vi "data logging.vi"   [LabVIEW 2017]
uses:
  Robot Global Data.vi
  <vilib>/Utility/file.llb/Write Delimited Spreadsheet (string).vi
types:
  T1 = typedef "WPI_EncoderDevRef.ctl" = cluster{"DevStatus":errorcluster, "EncoderIndex":T2, "CounterIndex":T3, "DistancePerCount":dbl, "Decoding Type":T4}
  T2 = typedef "FPGA_EncoderIdx.ctl" = enum8{"Enc 0", "Enc 1", "Enc 2", "Enc 3", "Enc 4", "Enc 5", "Enc 6", "Enc 7", "Invalid"}
  T3 = typedef "FPGA_CounterCtrSystemIndex.ctl" = enum8{"Ctr 0", "Ctr 1", "Ctr 2", "Ctr 3", "Ctr 4", "Ctr 5", "Ctr 6", "Ctr 7", "Invalid"}
  T4 = typedef "WPI_EncoderType.ctl" = enum16{"1x", "2x", "4x"}
  T5 = cluster{"Yaw":dbl, "Roll":dbl, "Pitch":dbl, "Heading":dbl, "Fused Heading":dbl}
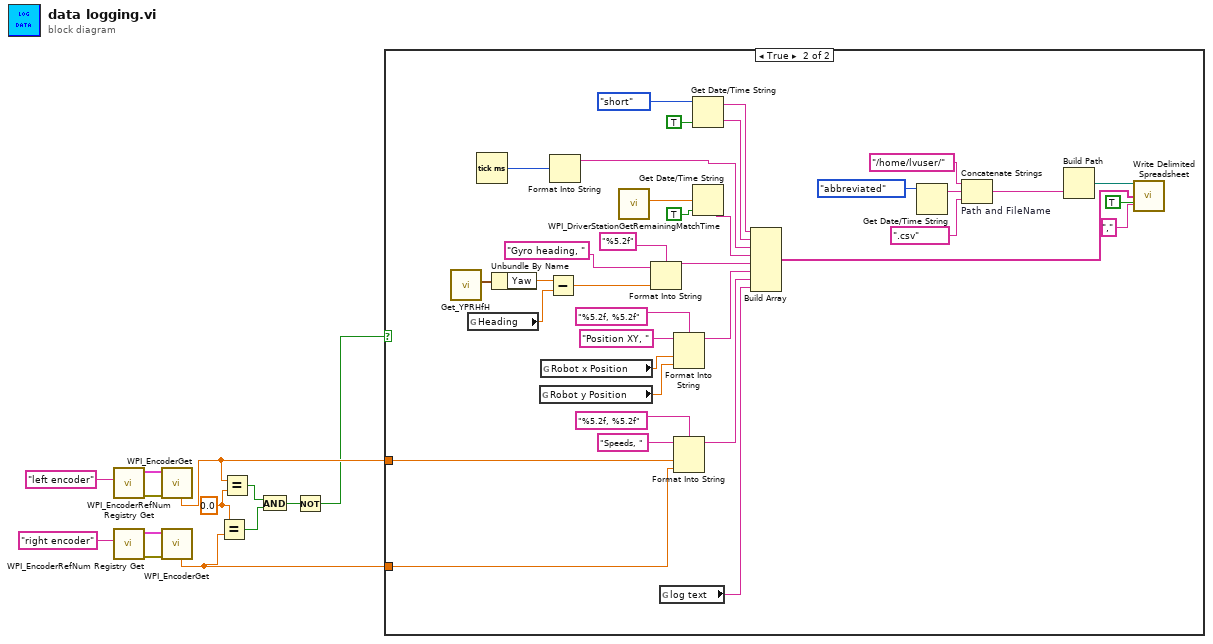
[diagram p0: block diagram]
diagram:
  w6 = 0.0 ("y")
  n1 = call <vilib>:"WPI_EncoderRefNum Registry Get.vi"("refnum name"="left encoder") -> ("error out"=w11:errorcluster, "EncoderDevRef"=w10:T1)  [unwired: 9 in]
  n2 = call <vilib>:"WPI_EncoderRefNum Registry Get.vi"("refnum name"="right encoder") -> ("error out"=w13:errorcluster, "EncoderDevRef"=w12:T1)  [unwired: 9 in]
  n3 = call <vilib>:"WPI_EncoderGet.vi"("error in (no error)"=w11, "EncoderDevRef"=w10) -> ("Rate"=w7:dbl)  [unwired: 4 in, 5 out]
  n4 = call <vilib>:"WPI_EncoderGet.vi"("error in (no error)"=w13, "EncoderDevRef"=w12) -> ("Rate"=w5:dbl)  [unwired: 4 in, 5 out]
  n5 = Equal?(x=w6, y=w5) -> (x = y?=w3:bool)
  n6 = Equal?(x=w7, y=w6) -> (x = y?=w4:bool)
  n7 = And(x=w4, y=w3) -> (x .and. y?=w2:bool)
  n8 = Not(x=w2) -> (.not. x?=w1:bool)
  n9 = case shown="True" w1 {
    tunnel: w7 -> [_ w15]
    tunnel: w5 -> [_ w14]
    frame False {
    }
    frame True {
      n10 = call <vilib>:"Get_YPRHfH.vi"() -> ("YRPHfH"=w41:T5)  [unwired: 11 in]
      n11 = global read "Robot Global Data.vi" "Heading"() -> (w49:dbl)
      n12 = Tick Count (ms)() -> (millisecond timer value=w17:u32)
      n13 = Unbundle By Name(w41) -> ("Yaw"=w42:dbl)
      n14 = global read "Robot Global Data.vi" "Robot y Position"() -> (w24:dbl)
      n15 = global read "Robot Global Data.vi" "Robot x Position"() -> (w32:dbl)
      n16 = Subtract(x=w42, y=w49) -> (x-y=w39:dbl)
      n17 = Format Into String(w17) -> (resulting string=w16:string)  [unwired: 3 in, 1 out]
      n18 = call <vilib>:"WPI_DriverStationGetRemainingMatchTime.vi"() -> ("Match Time(s)"=w48:sgl)  [unwired: 10 in, 1 out]
      n19 = Format Into String(format string="%5.2f", initial string="Gyro heading, " ("element"), w39) -> (resulting string=w21:string)  [unwired: 1 in, 1 out]
      n20 = global read "Robot Global Data.vi" "log text"() -> (w18:string)
      n21 = Format Into String(format string="%5.2f, %5.2f", initial string="Position XY, ", w32, w24) -> (resulting string=w20:string)  [unwired: 1 in, 1 out]
      n22 = Format Into String(format string="%5.2f, %5.2f", initial string="Speeds, ", w15, w14) -> (resulting string=w19:string)  [unwired: 1 in, 1 out]
      n23 = Get Date/Time String(date format (0)=enum16{"short", "long", "abbreviated"}."short", want seconds? (F)=TRUE) -> (date string=w31:string, time string=w30:string)  [unwired: 1 in]
      n24 = Get Date/Time String(seconds (now)=w48, want seconds? (F)=TRUE) -> (time string=w43:string)  [unwired: 1 in, 1 out]
      n25 = Build Array(w31, w30, w16, w43, w21, w20, w19, w18) -> (w46:string[])
      n26 = Get Date/Time String(date format (0)=enum16{"short", "long", "abbreviated"}."abbreviated") -> (date string=w33:string)  [unwired: 2 in, 1 out]
      n27 = Concatenate Strings "Path and FileName"("/home/lvuser/", w33, ".csv") -> (w36:string)
      n28 = Build Path(name or relative path=w36) -> (appended path=w35:path)  [unwired: 1 in]
      n29 = call-poly <vilib>:"Write Delimited Spreadsheet.vi"("file path (dialog if empty)"=w35, "1D data"=w46, "append to file? (new file:F)"=TRUE, "delimiter (\\t)"="," ("delimiter (\\t)")) -> ()  [unwired: 10 in, 2 out]
    }
  }
